vi "Excel_Report.vi"(5 "Language":T1, 6 "Process":refnum<vi>, 7 "Report":T2, 8 "error in":errorcluster, 9 "Backup path":path, 10 "Report path":path, 11 "template (empty)":path) -> (0 "error out":errorcluster, 2 "Message":string)   [LabVIEW 2015]
doc: "输出打印报表"
uses:
  CustomControl/Report Info.ctl
  CustomControl/ReportTitle.ctl
  CustomControl/Lang_Control.ctl
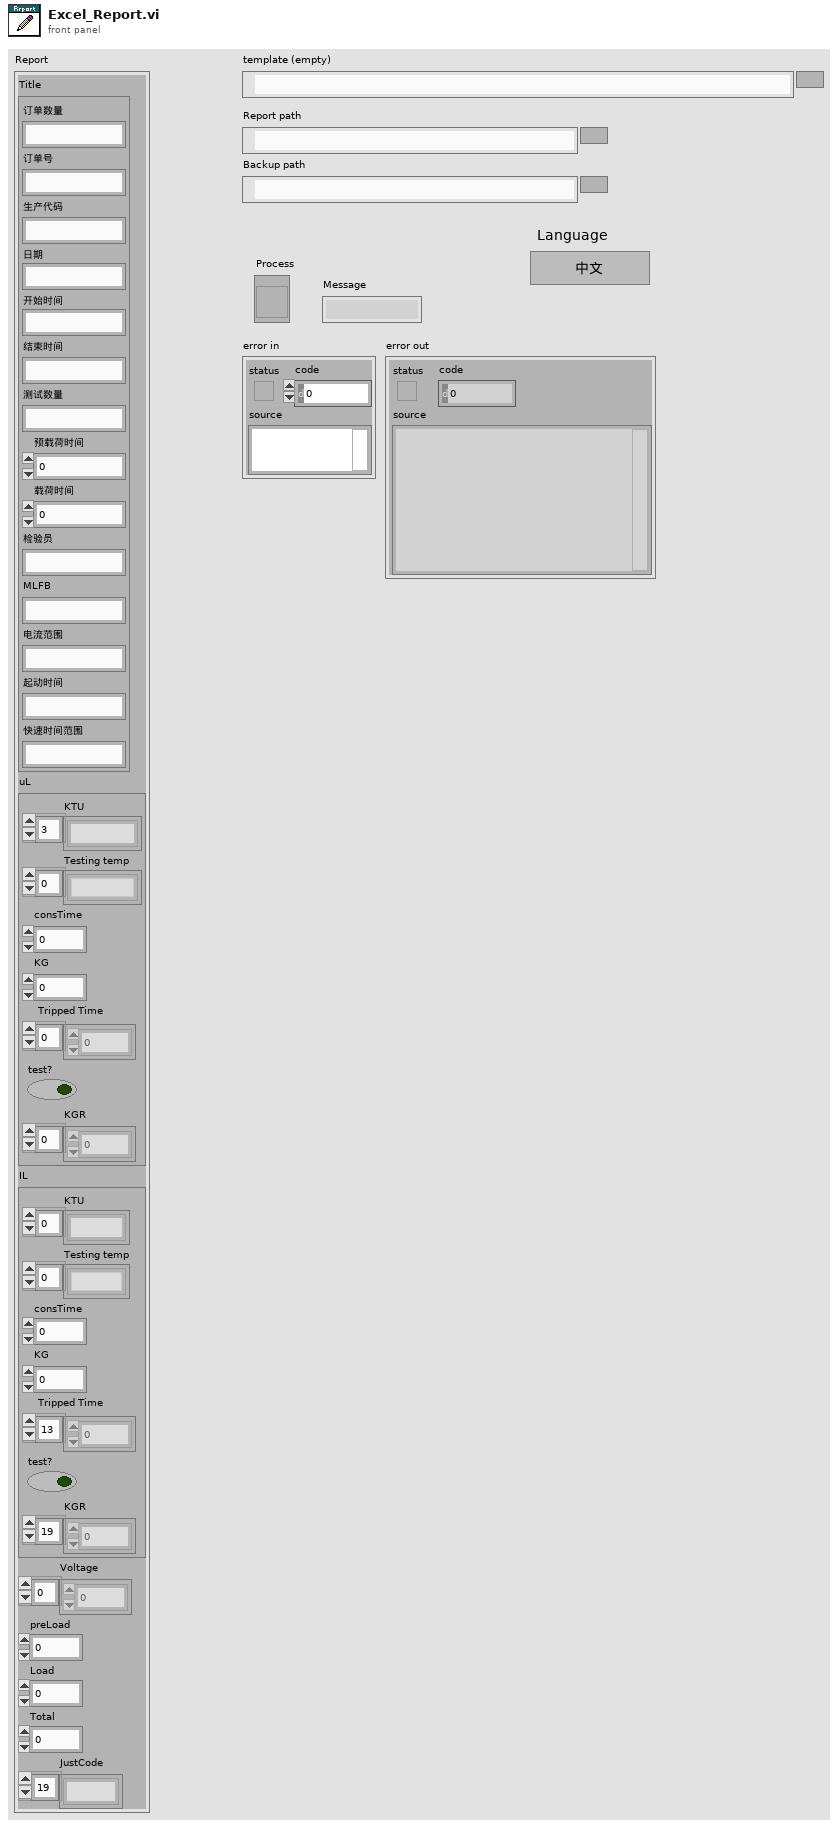
[diagram p1: front panel]
types:
  T1 = typedef "Lang_Control.ctl" = enum16{"中文", "English"}
  T2 = typedef "Report Info.ctl" = cluster{"Title":T3, "uL":cluster{"KTU":string[], "Testing temp":string[], "consTime":i32, "KG":dbl, "Tripped Time":i32[], "test?":bool, "KGR":dbl[]}, "IL":cluster{"KTU":string[], "Testing temp":string[], "consTime":i32, "KG":dbl, "Tripped Time":i32[], "test?":bool, "KGR":dbl[]}, "Voltage":dbl[], "preLoad":i32, "Load":i32, "Total":i32, "JustCode":string[]}
  T3 = typedef "ReportTitle.ctl" = cluster{"订单数量":string, "订单号":string, "生产代码":string, "日期":string, "开始时间":string, "结束时间":string, "测试数量":string, "预载荷时间":i32, "载荷时间":i32, "检验员":string, "MLFB":string, "电流范围":string, "起动时间":string, "快速时间范围":string}
  T4 = cluster{"KG20":string[], "temperature":string[], "consTime":i32, "KG":dbl}
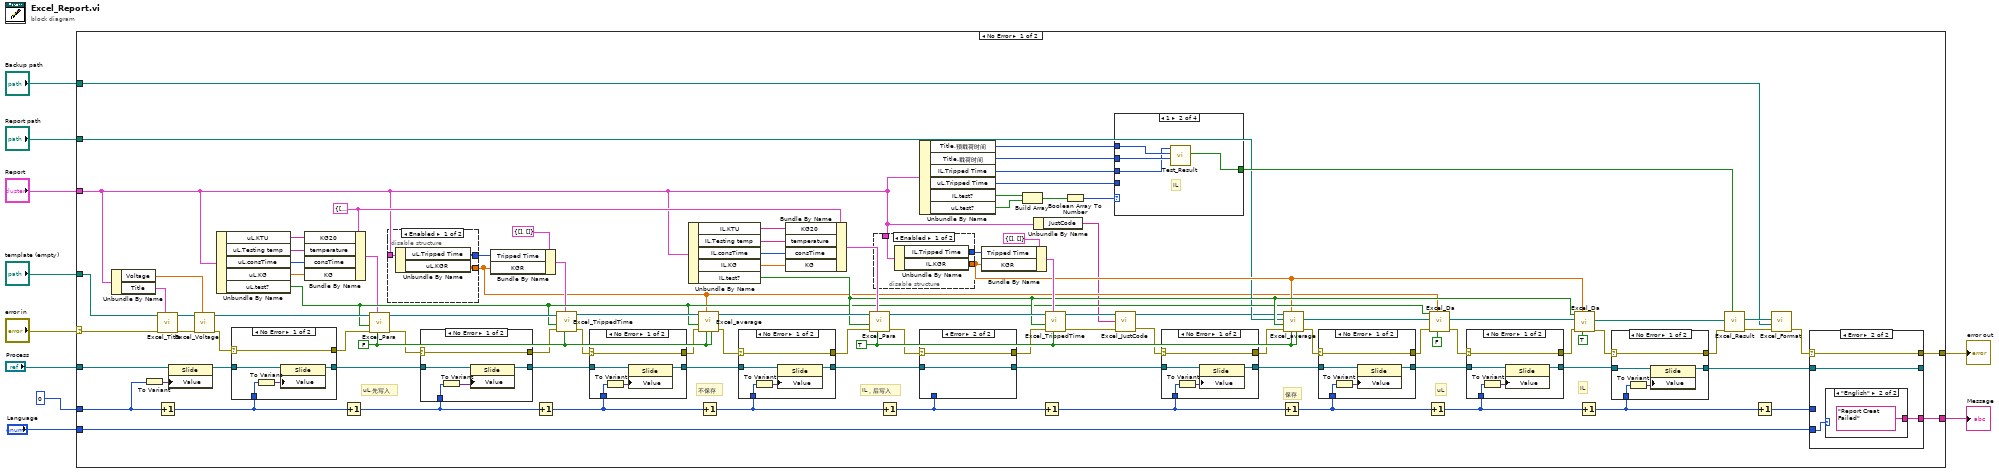
[diagram p0: block diagram]
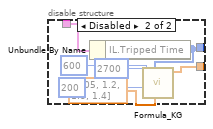
[diagram p2: hidden frame]
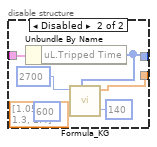
[diagram p3: hidden frame]
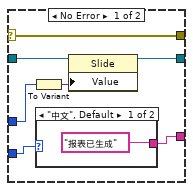
[diagram p4: hidden frame]
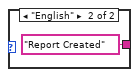
[diagram p5: hidden frame]
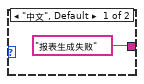
[diagram p6: hidden frame]
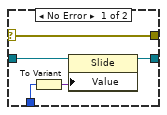
[diagram p11: hidden frame]
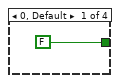
[diagram p16: hidden frame]
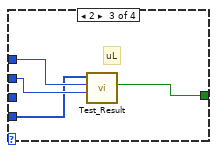
[diagram p17: hidden frame]
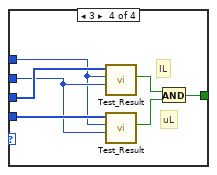
[diagram p18: hidden frame]
diagram:
  n1 = case shown="No Error" "error in" {
    selector: "error in" -> [w37 w227]
    tunnel: "template (empty)" -> [w111 _]
    tunnel: "Report" -> [w12 _]
    tunnel: "Process" -> [w22 _]
    tunnel: [w39 w227] -> w8
    tunnel: "Report path" -> [w36 _]
    tunnel: "Backup path" -> [w35 _]
    tunnel: "Language" -> [w34 _]
    tunnel: [w33 _] -> w3
    tunnel: 0 -> [w19 _]
    frame No Error {
      w66 = T4 {"KG20"=[], "temperature"=[], "consTime"=0, "KG"=0.0} ("Test parameter")
      w69 = TRUE
      w71 = FALSE ("1_IL,0_uL")
      # "保存"
      # "不保存"
      # "IL"
      # "uL"
      # "uL,先写入"
      # "IL，后写入"
      n2 = Unbundle By Name(w12) -> ("Voltage"=w76:dbl[], "Title"=w77:T3)
      n3 = To Variant(anything=w19) -> (Variant=w20:variant)
      n4 = call "Excel_Title.vi"("Report_Title"=w77, "error in (no error)"=w37, "Template path"=w111) -> ("error out"=w112:errorcluster, "report out"=w88:refnum<class "NI_report.lvclass">)  [unwired: 6 in, 1 out]
      n5 = Increment(x=w19) -> (x+1=w32:i32)
      n6 = property class="Slide"(reference=w22, "Value"=w20) -> (reference out=w21:refnum<vi>)  [unwired: 1 in, 1 out]
      n7 = call "Excel_Voltage.vi"("duanVoltage"=w76, "error in (no error)"=w112, "report in"=w88) -> ("error out"=w65:errorcluster, "report out"=w87:refnum<class "NI_report.lvclass">)  [unwired: 6 in, 1 out]
      n8 = Unbundle By Name(w12) -> ("uL.KTU"=w105:string[], "uL.Testing temp"=w104:string[], "uL.consTime"=w103:i32, "uL.KG"=w74:dbl, "uL.test?"=w80:bool)
      n9 = case shown="No Error" w65 {
        selector: w65 -> [w208 w210]
        tunnel: [w208 w210] -> w64
        tunnel: w21 -> [w207 w209]
        tunnel: [w205 w209] -> w61
        tunnel: w32 -> [w204 _]
        frame No Error {
          n10 = To Variant(anything=w204) -> (Variant=w206:variant)
          n11 = property class="Slide"(reference=w207, "Value"=w206) -> (reference out=w205:refnum<vi>)  [unwired: 1 in, 1 out]
        }
        frame Error {
        }
      }
      n12 = Bundle By Name(cluster=w66, "KG20"=w105, "temperature"=w104, "consTime"=w103, "KG"=w74) -> (w75:T4)
      n13 = Increment(x=w32) -> (x+1=w31:i32)
      n14 = call "Excel_Para.vi"("1_IL,0_uL"=w71, "Test parameter"=w75, "error in (no error)"=w64, "Test?"=w80, "report in"=w87) -> ("error out"=w63:errorcluster, "report out"=w86:refnum<class "NI_report.lvclass">)  [unwired: 4 in, 1 out]
      n15 = disable-structure shown="Enabled" {
        disable-tunnel: [w125 w131] -> w18
        disable-tunnel: [w124 w130] -> w17
        disable-tunnel: w12 -> [w123 w132]
        frame Enabled {
          n16 = Unbundle By Name(w123) -> ("uL.Tripped Time"=w125:i32[], "uL.KGR"=w124:dbl[])
        }
        frame Disabled {
          n17 = Unbundle By Name(w132) -> ("uL.Tripped Time"=w131:i32[])
          n18 = call "Formula_KG.vi"("KTu"=dbl[] [1.05, 1.2, 1.3, 1.4], "Tripped Time"=w131, "consTime"=140, "Load Time"=600, "Preload Time"=2700) -> ("KGR"=w130:dbl[])  [unwired: 5 in, 1 out]
        }
      }
      n19 = case shown="No Error" w63 {
        selector: w63 -> [w201 w203]
        tunnel: [w201 w203] -> w62
        tunnel: w61 -> [w200 w202]
        tunnel: [w198 w202] -> w58
        tunnel: w31 -> [w197 _]
        frame No Error {
          n20 = To Variant(anything=w197) -> (Variant=w199:variant)
          n21 = property class="Slide"(reference=w200, "Value"=w199) -> (reference out=w198:refnum<vi>)  [unwired: 1 in, 1 out]
        }
        frame Error {
        }
      }
      n22 = Bundle By Name(cluster=cluster{"Tripped Time":i32[], "KGR":dbl[]} {"Tripped Time"=[], "KGR"=[]} ("Result"), "Tripped Time"=w18, "KGR"=w17) -> (w72:cluster{"Tripped Time":i32[], "KGR":dbl[]})
      n23 = Increment(x=w31) -> (x+1=w30:i32)
      n24 = call "Excel_TrippedTime.vi"("1_IL,0_uL"=w71, "Result"=w72, "error in (no error)"=w62, "Test?"=w80, "report in"=w86) -> ("error out"=w60:errorcluster, "report out"=w89:refnum<class "NI_report.lvclass">)  [unwired: 4 in, 1 out]
      n25 = case shown="No Error" w60 {
        selector: w60 -> [w194 w196]
        tunnel: [w194 w196] -> w59
        tunnel: w58 -> [w193 w195]
        tunnel: [w191 w195] -> w55
        tunnel: w30 -> [w190 _]
        frame No Error {
          n26 = To Variant(anything=w190) -> (Variant=w192:variant)
          n27 = property class="Slide"(reference=w193, "Value"=w192) -> (reference out=w191:refnum<vi>)  [unwired: 1 in, 1 out]
        }
        frame Error {
        }
      }
      n28 = Unbundle By Name(w12) -> ("IL.KTU"=w99:string[], "IL.Testing temp"=w100:string[], "IL.consTime"=w101:i32, "IL.KG"=w102:dbl, "IL.test?"=w81:bool)
      n29 = call "Excel_average.vi"("Save?"=w71, "1_IL,0_uL"=w71, "KG20"=w17, "error in (no error)"=w59, "Test?"=w80, "report in"=w89) -> ("error out"=w57:errorcluster, "report out"=w83:refnum<class "NI_report.lvclass">)  [unwired: 3 in, 1 out]
      n30 = Increment(x=w30) -> (x+1=w29:i32)
      n31 = case shown="No Error" w57 {
        selector: w57 -> [w187 w189]
        tunnel: [w187 w189] -> w56
        tunnel: w55 -> [w186 w188]
        tunnel: [w184 w188] -> w52
        tunnel: w29 -> [w183 _]
        frame No Error {
          n32 = To Variant(anything=w183) -> (Variant=w185:variant)
          n33 = property class="Slide"(reference=w186, "Value"=w185) -> (reference out=w184:refnum<vi>)  [unwired: 1 in, 1 out]
        }
        frame Error {
        }
      }
      n34 = Bundle By Name(cluster=w66, "KG20"=w99, "temperature"=w100, "consTime"=w101, "KG"=w102) -> (w98:T4)
      n35 = call "Excel_Para.vi"("1_IL,0_uL"=w69, "Test parameter"=w98, "error in (no error)"=w56, "Test?"=w81, "report in"=w83) -> ("error out"=w54:errorcluster, "report out"=w85:refnum<class "NI_report.lvclass">)  [unwired: 4 in, 1 out]
      n36 = disable-structure shown="Enabled" {
        disable-tunnel: [w115 w121] -> w96
        disable-tunnel: [w114 w120] -> w67
        disable-tunnel: w12 -> [w113 w122]
        frame Enabled {
          n37 = Unbundle By Name(w113) -> ("IL.Tripped Time"=w115:i32[], "IL.KGR"=w114:dbl[])
        }
        frame Disabled {
          n38 = Unbundle By Name(w122) -> ("IL.Tripped Time"=w121:i32[])
          n39 = call "Formula_KG.vi"("KTu"=dbl[] [1.05, 1.2, 1.3, 1.4], "Tripped Time"=w121, "consTime"=200, "Load Time"=600, "Preload Time"=2700) -> ("KGR"=w120:dbl[])  [unwired: 5 in, 1 out]
        }
      }
      n40 = Increment(x=w29) -> (x+1=w28:i32)
      n41 = Unbundle By Name(w12) -> ("Title.预载荷时间"=w93:i32, "Title.载荷时间"=w92:i32, "IL.Tripped Time"=w91:i32[], "uL.Tripped Time"=w90:i32[], "IL.test?"=w95:bool, "uL.test?"=w94:bool)
      n42 = case shown="Error" w54 {
        selector: w54 -> [w180 w182]
        tunnel: [w180 w182] -> w53
        tunnel: w52 -> [w179 w181]
        tunnel: [w177 w181] -> w50
        tunnel: w28 -> [w176 _]
        frame No Error {
          n43 = To Variant(anything=w176) -> (Variant=w178:variant)
          n44 = property class="Slide"(reference=w179, "Value"=w178) -> (reference out=w177:refnum<vi>)  [unwired: 1 in, 1 out]
        }
        frame Error {
        }
      }
      n45 = Bundle By Name(cluster=cluster{"Tripped Time":i32[], "KGR":dbl[]} {"Tripped Time"=[], "KGR"=[]} ("Result"), "Tripped Time"=w96, "KGR"=w67) -> (w97:cluster{"Tripped Time":i32[], "KGR":dbl[]})
      n46 = Build Array(w95, w94) -> (w109:bool[])
      n47 = Unbundle By Name(w12) -> ("JustCode"=w11:string[])
      n48 = Increment(x=w28) -> (x+1=w27:i32)
      n49 = call "Excel_TrippedTime.vi"("1_IL,0_uL"=w69, "Result"=w97, "error in (no error)"=w53, "Test?"=w81, "report in"=w85) -> ("error out"=w13:errorcluster, "report out"=w16:refnum<class "NI_report.lvclass">)  [unwired: 4 in, 1 out]
      n50 = Boolean Array To Number(Boolean array=w109) -> (number=w108:u32)
      n51 = case shown="1" w108 {
        tunnel: [FALSE w215 w219 w224] -> w110
        tunnel: w93 -> [_ w214 w217 w220]
        tunnel: w92 -> [_ w213 w218 w221]
        tunnel: w91 -> [_ w212 _ w223]
        tunnel: w90 -> [_ _ w216 w222]
        frame 0, Default {
        }
        frame 1 {
          # "IL"
          n52 = call "Test_Result.vi"("Load Time"=w213, "Preload Time"=w214, "Tripped Time"=w212) -> ("Pass/Fail?"=w215:bool)  [unwired: 8 in]
        }
        frame 2 {
          # "uL"
          n53 = call "Test_Result.vi"("Load Time"=w218, "Preload Time"=w217, "Tripped Time"=w216) -> ("Pass/Fail?"=w219:bool)  [unwired: 8 in]
        }
        frame 3 {
          # "IL"
          # "uL"
          n54 = call "Test_Result.vi"("Load Time"=w221, "Preload Time"=w220, "Tripped Time"=w223) -> ("Pass/Fail?"=w225:bool)  [unwired: 8 in]
          n55 = call "Test_Result.vi"("Load Time"=w221, "Preload Time"=w220, "Tripped Time"=w222) -> ("Pass/Fail?"=w226:bool)  [unwired: 8 in]
          n56 = And(x=w225, y=w226) -> (x .and. y?=w224:bool)
        }
      }
      n57 = call "Excel_JustCode.vi"("error in (no error)"=w13, "JustCode"=w11, "report in"=w16) -> ("error out"=w14:errorcluster, "report out"=w15:refnum<class "NI_report.lvclass">)  [unwired: 1 in]
      n58 = case shown="No Error" w14 {
        selector: w14 -> [w173 w175]
        tunnel: [w173 w175] -> w51
        tunnel: w50 -> [w172 w174]
        tunnel: [w170 w174] -> w47
        tunnel: w27 -> [w169 _]
        frame No Error {
          n59 = To Variant(anything=w169) -> (Variant=w171:variant)
          n60 = property class="Slide"(reference=w172, "Value"=w171) -> (reference out=w170:refnum<vi>)  [unwired: 1 in, 1 out]
        }
        frame Error {
        }
      }
      n61 = Increment(x=w27) -> (x+1=w26:i32)
      n62 = call "Excel_average.vi"("Save?"=w69, "1_IL,0_uL"=w69, "KG20"=w67, "error in (no error)"=w51, "Test?"=w81, "Report path in"=w36, "report in"=w15) -> ("error out"=w49:errorcluster, "Report path out"=w79:path)  [unwired: 2 in, 1 out]
      n63 = case shown="No Error" w49 {
        selector: w49 -> [w166 w168]
        tunnel: [w166 w168] -> w48
        tunnel: w47 -> [w165 w167]
        tunnel: [w163 w167] -> w44
        tunnel: w26 -> [w162 _]
        frame No Error {
          n64 = To Variant(anything=w162) -> (Variant=w164:variant)
          n65 = property class="Slide"(reference=w165, "Value"=w164) -> (reference out=w163:refnum<vi>)  [unwired: 1 in, 1 out]
        }
        frame Error {
        }
      }
      n66 = Increment(x=w26) -> (x+1=w25:i32)
      n67 = call "Excel_Da.vi"("(1_IL,0_uL)"=FALSE, "KG20"=w17, "error in (no error)"=w48, "Report path in"=w79, "Test?"=w80) -> ("error out"=w46:errorcluster, "Report path out"=w78:path)  [unwired: 5 in]
      n68 = case shown="No Error" w46 {
        selector: w46 -> [w159 w161]
        tunnel: [w159 w161] -> w45
        tunnel: w44 -> [w158 w160]
        tunnel: [w156 w160] -> w41
        tunnel: w25 -> [w155 _]
        frame No Error {
          n69 = To Variant(anything=w155) -> (Variant=w157:variant)
          n70 = property class="Slide"(reference=w158, "Value"=w157) -> (reference out=w156:refnum<vi>)  [unwired: 1 in, 1 out]
        }
        frame Error {
        }
      }
      n71 = call "Excel_Da.vi"("(1_IL,0_uL)"=TRUE, "KG20"=w67, "error in (no error)"=w45, "Report path in"=w78, "Test?"=w81) -> ("error out"=w43:errorcluster, "Report path out"=w82:path)  [unwired: 5 in]
      n72 = Increment(x=w25) -> (x+1=w24:i32)
      n73 = case shown="No Error" w43 {
        selector: w43 -> [w152 w154]
        tunnel: [w152 w154] -> w42
        tunnel: w41 -> [w151 w153]
        tunnel: [w149 w153] -> w38
        tunnel: w24 -> [w148 _]
        frame No Error {
          n74 = To Variant(anything=w148) -> (Variant=w150:variant)
          n75 = property class="Slide"(reference=w151, "Value"=w150) -> (reference out=w149:refnum<vi>)  [unwired: 1 in, 1 out]
        }
        frame Error {
        }
      }
      n76 = call "Excel_Result.vi"("Pass/Fail"=w110, "error in (no error)"=w42, "Report path in"=w82) -> ("error out"=w106:errorcluster, "Report path out"=w107:path)  [unwired: 7 in]
      n77 = Increment(x=w24) -> (x+1=w23:i32)
      n78 = call "Excel_Format.vi"("error in (no error)"=w106, "Backup path"=w35, "file path"=w107) -> ("error out"=w40:errorcluster)  [unwired: 8 in]
      n79 = case shown="Error" w40 {
        selector: w40 -> [w139 w145]
        tunnel: [w139 w145] -> w39
        tunnel: w38 -> [w138 w144]
        tunnel: [w136 w144] -> _
        tunnel: w34 -> [w135 w143]
        tunnel: [w134 w142] -> w33
        tunnel: w23 -> [w133 _]
        frame No Error {
          n80 = To Variant(anything=w133) -> (Variant=w137:variant)
          n81 = case shown="\"中文\", Default" w135 {
            tunnel: ["报表已生成" "Report Created"] -> w134
            frame "中文", Default {
            }
            frame "English" {
            }
          }
          n82 = property class="Slide"(reference=w138, "Value"=w137) -> (reference out=w136:refnum<vi>)  [unwired: 1 in, 1 out]
        }
        frame Error {
          n83 = case shown="\"English\"" w143 {
            tunnel: ["报表生成失败" "Report Creat Failed"] -> w142
            frame "中文", Default {
            }
            frame "English" {
            }
          }
        }
      }
    }
    frame Error {
    }
  }
  "error out" <- w8
  "Message" <- w3
